vi "Sample_Data_Subset.vi"(11 "Particle Measurements (Pixels)":dbl[][](array[numeric]) format="%.2f") -> (3 "Sample Data":dbl[](array[numeric]))   [LabVIEW 2022 SP3]
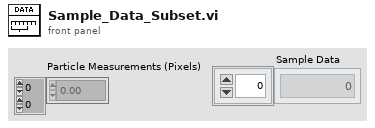
[diagram p1: front panel]
types:
  T1 = typedef "Particle Parameters" = i32
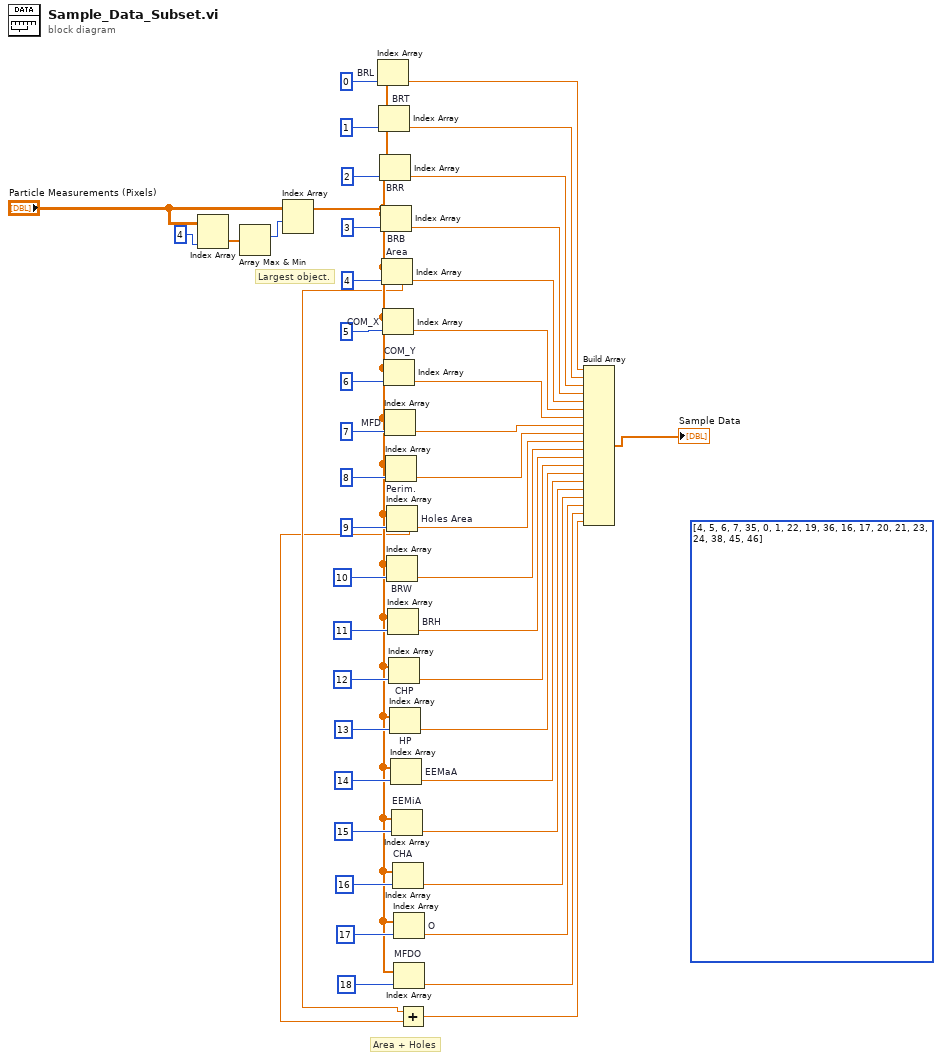
[diagram p0: block diagram]
diagram:
  (unwired) T1[] [4, 5, 6, 7, 35, 0, 1, 22, 19, 36, 16, 17, 20, 21, 23, 24, 38, 45, 46] items=["Center of Mass X", "Center of Mass Y", "First Pixel X", "First Pixel Y", "Bounding Rect Left", "Bounding Rect Top", "Bounding Rect Right", "Bounding Rect Bottom", "Max Feret Diameter Start X", "Max Feret Diameter Start Y", "Max Feret Diameter End X", "Max Feret Diameter End Y", "Max Horiz. Segment Length Left", "Max Horiz. Segment Length Right", "Max Horiz. Segment Length Row", "-", "Bounding Rect Width", "Bounding Rect Height", "Bounding Rect Diagonal", "Perimeter", "Convex Hull Perimeter", "Holes' Perimeter", "Max Feret Diameter", "Equivalent Ellipse Major Axis", "Equivalent Ellipse Minor Axis", "Equivalent Ellipse Minor Axis (Feret)", "Equivalent Rect Long Side", "Equivalent Rect Short Side", "Equivalent Rect Diagonal", "Equivalent Rect Short Side (Feret)", "Average Horiz. Segment Length", "Average Vert. Segment Length", "Hydraulic Radius", "Waddel Disk Diameter", "-", "Area", "Holes' Area", "Particle & Holes' Area", "Convex Hull Area", "Image Area", "-", "Number of Holes", "Number of Horiz. Segments", "Number of Vert. Segments", "-", "Orientation", "Max Feret Diameter Orientation", "-", "% Area/Image Area", "% Area/(Particle & Holes' Area)", "Ratio of Equivalent Ellipse Axes", "Ratio of Equivalent Rect Sides", "-", "Elongation Factor", "Compactness Factor", "Heywood Circularity Factor", "Type Factor", "-", "Sum X", "Sum Y", "Sum XX", "Sum XY", "Sum YY", "Sum XXX", "Sum XXY", "Sum XYY", "Sum YYY", "-", "Moment of Inertia XX", "Moment of Inertia XY", "Moment of Inertia YY", "Moment of Inertia XXX", "Moment of Inertia XXY", "Moment of Inertia XYY", "Moment of Inertia YYY", "Norm. Moment of Inertia XX", "Norm. Moment of Inertia XY", "Norm. Moment of Inertia YY", "Norm. Moment of Inertia XXX", "Norm. Moment of Inertia XXY", "Norm. Moment of Inertia XYY", "Norm. Moment of Inertia YYY", "Hu Moment 1", "Hu Moment 2", "Hu Moment 3", "Hu Moment 4", "Hu Moment 5", "Hu Moment 6", "Hu Moment 7"] ("Pixel Measurements")
  # "Area + Holes"
  # "Largest object."
  n1 = Index Array(array="Particle Measurements (Pixels)", index (col)=4 ("index (row)")) -> (element=w43:dbl[])  [unwired: 1 in]
  n2 = Array Max & Min(array=w43) -> (max index (indices)=w44:i32)  [unwired: 3 out]
  n3 = Index Array(array="Particle Measurements (Pixels)", index (row)=w44) -> (element=w22:dbl[])  [unwired: 1 in]
  n4 = Index Array "BRL"(array=w22, index=0) -> (element=w20:dbl)
  n5 = Index Array "BRT"(array=w22, index=1) -> (element=w19:dbl)
  n6 = Index Array "BRR"(array=w22, index=2) -> (element=w18:dbl)
  n7 = Index Array "BRB"(array=w22, index=3) -> (element=w17:dbl)
  n8 = Index Array "Area"(array=w22, index=4) -> (element=w16:dbl)
  n9 = Index Array "COM_X"(array=w22, index=5) -> (element=w15:dbl)
  n10 = Index Array "COM_Y"(array=w22, index=6) -> (element=w14:dbl)
  n11 = Index Array "MFD"(array=w22, index=7) -> (element=w13:dbl)
  n12 = Index Array "Perim."(array=w22, index=8) -> (element=w12:dbl)
  n13 = Index Array "Holes Area"(array=w22, index=9) -> (element=w11:dbl)
  n14 = Index Array "BRW"(array=w22, index=10) -> (element=w10:dbl)
  n15 = Index Array "BRH"(array=w22, index=11) -> (element=w9:dbl)
  n16 = Index Array "CHP"(array=w22, index=12) -> (element=w8:dbl)
  n17 = Index Array "HP"(array=w22, index=13) -> (element=w7:dbl)
  n18 = Index Array "EEMaA"(array=w22, index=14) -> (element=w6:dbl)
  n19 = Index Array "EEMiA"(array=w22, index=15) -> (element=w5:dbl)
  n20 = Index Array "CHA"(array=w22, index=16) -> (element=w4:dbl)
  n21 = Index Array "O"(array=w22, index=17) -> (element=w3:dbl)
  n22 = Index Array "MFDO"(array=w22, index=18) -> (element=w2:dbl)
  n23 = Add(x=w16, y=w11) -> (x+y=w1:dbl)
  n24 = Build Array(w20, w19, w18, w17, w16, w15, w14, w13, w12, w11, w10, w9, w8, w7, w6, w5, w4, w3, w2, w1) -> (→"Sample Data":dbl[])
